vi "Get Serial Number.vi"(0 "COM Port in":refnum<visa-resource-name>, 1 "error in":errorcluster) -> (2 "COM Port out":refnum<visa-resource-name>, 3 "S/N":string, 4 "OK":bool, 5 "error out":errorcluster)   [LabVIEW 2013]
doc: "This command queries the serial number of the controller. The serial number needs to be\ninterpreted as a string. It may contain special characters like / or §.\nThe serial number is for informative use only.\n\nThe PhoxXR lasers have the controller separated from the laser head. This command\nqueries the controller data which is the main device data. The laser heads serial\nnumber for PhoxXR lasers can be queried with the command ?GSH"
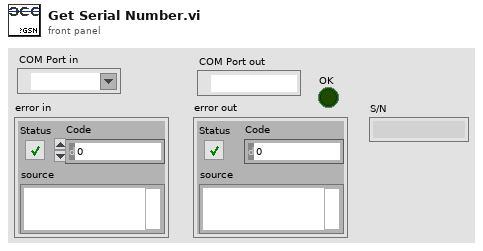
[diagram p1: front panel]
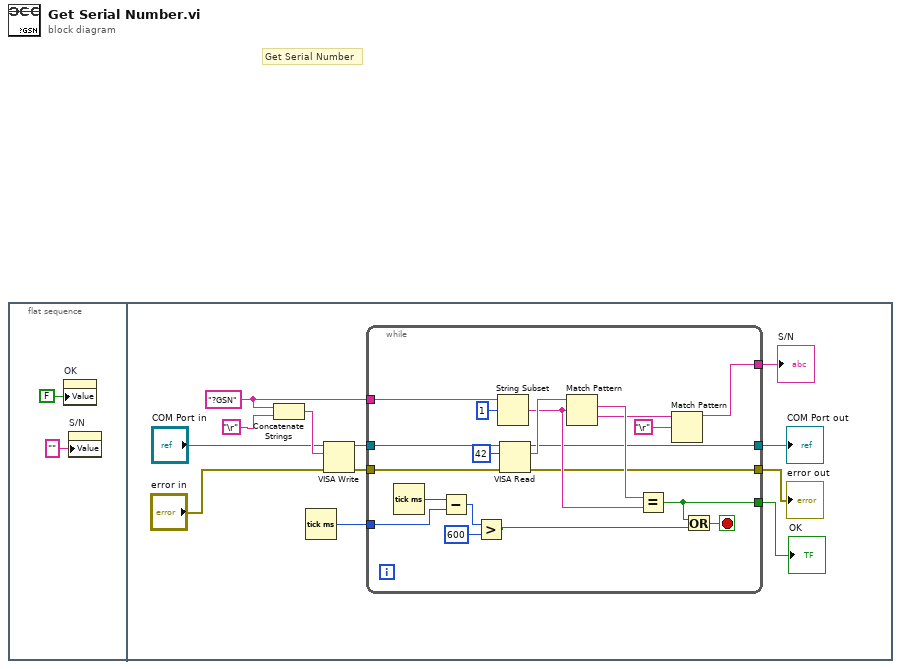
[diagram p0: block diagram]
diagram:
  # "Get Serial Number"
  n1 = flat-sequence {
    frame #0 {
      n2 = property on="OK" class="Bool. (strikt)"("Value"=FALSE ("OK")) -> ()  [unwired: 2 in, 2 out]
      n3 = property on="S/N" class="Str"("Value"="" ("S/N")) -> ()  [unwired: 2 in, 2 out]
    }
    frame #1 {
      w5 = "?GSN" ("Schreibpuffer")
      n4 = Concatenate Strings(w5, "\r") -> (w11:string)
      n5 = Tick Count (ms)() -> (millisecond timer value=w3:u32)
      n6 = VISA Write(VISA resource name="COM Port in", write buffer=w11, error in (no error)="error in") -> (VISA resource name out=w9:refnum<visa-resource-name>, error out=w8:errorcluster)  [unwired: 1 out]
      n7 = while {
        tunnel: [w29] -> w14
        tunnel: [w28] -> w13
        tunnel: [w27] -> w12
        tunnel: w9 -> [w21]
        tunnel: w8 -> [w24]
        tunnel: w5 -> [w23]
        tunnel: [w22] -> w4
        tunnel: w3 -> [w16]
        stop <- w25 stop-if-true
        n8 = Tick Count (ms)() -> (millisecond timer value=w18:u32)
        n9 = Subtract(x=w18, y=w16) -> (x-y=w19:u32)
        n10 = Greater?(x=w19, y=u32 600) -> (0:w17:bool)
        n11 = String Subset(string=w23, offset (0)=1 ("Offset (0)")) -> (substring=w30:string)  [unwired: 1 in]
        n12 = VISA Read(VISA resource name=w21, byte count=u32 42 ("Byte-Anzahl"), error in (no error)=w24) -> (VISA resource name out=w29:refnum<visa-resource-name>, read buffer=w33:string, error out=w28:errorcluster)  [unwired: 1 out]
        n13 = Match Pattern(string=w33, regular expression=w30) -> (match substring=w32:string, after substring=w26:string)  [unwired: 1 in, 2 out]
        n14 = Equal?(x=w32, y=w30) -> (x = y?=w22:bool)
        n15 = Match Pattern(string=w26, regular expression="\r") -> (before substring=w27:string)  [unwired: 1 in, 3 out]
        n16 = Or(x=w22, y=w17) -> (x .or. y?=w25:bool)
      }
      "COM Port out" <- w14
      "error out" <- w13
      "S/N" <- w12
      "OK" <- w4
    }
  }
